vi "Close.vi"(8 "error in (no error)":errorcluster, 11 "PythonWrapper in":refnum<class "PythonWrapper.lvclass">) -> (0 "error out":errorcluster, 3 "PythonWrapper out":refnum<class "PythonWrapper.lvclass">)   [LabVIEW 2022 SP3, in "PythonWrapper.lvlib" / "PythonWrapper.lvclass"]
uses:
  PythonWrapper.lvclass
  PythonWrapper.lvclass/PythonWrapper.ctl
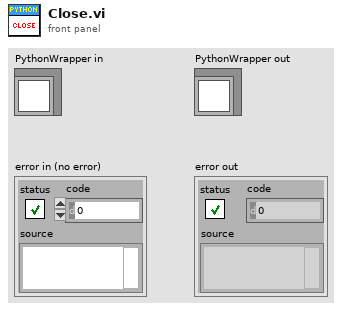
[diagram p1: front panel]
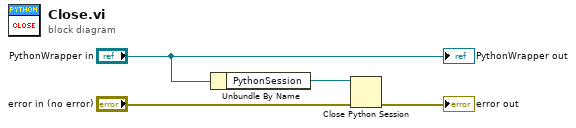
[diagram p0: block diagram]
diagram:
  n1 = Unbundle By Name("PythonWrapper in") -> ("PythonSession"=w3:refnum<k35>)
  n2 = Close Python Session(session in=w3, error in="error in (no error)") -> (11:→"error out":errorcluster)
  "PythonWrapper out" <- "PythonWrapper in"
